vi "Adjust Min-Max.vi"(7 "log?":bool, 8 "error in (no error)":errorcluster, 9 "Secondary Graph":refnum<vi>, 10 "Primary Graph":refnum<vi>, 11 "Scan Driver.lvclass":refnum<class "Scan Driver.lvclass">) -> (0 "error out":errorcluster, 2 "High":dbl, 3 "Scan Driver.lvclass out":refnum<class "Scan Driver.lvclass">)   [LabVIEW 2012, in "Scan Driver.lvclass"]
doc: "Set the boundaries of the onscreen scan graphs according to the extrema of the data store."
uses:
  Scan Driver.lvclass
  Scan Driver.lvclass/Scan Driver.ctl
  Scanners/Scanner/Scanner.lvclass
  File IO/File IO.lvclass
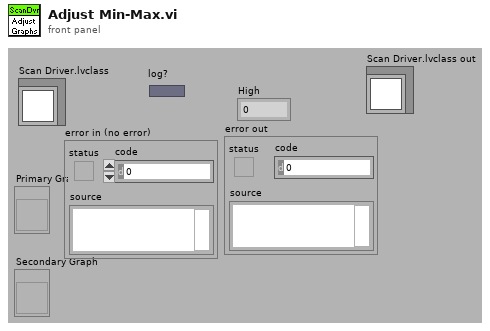
[diagram p1: front panel]
types:
  T1 = typedef "Readable.lvclass/Data Store.ctl" = T2[][]
  T2 = typedef "Readable.lvclass/Data Point.ctl" = cluster{"t":T3, "x":T4}
  T3 = typedef "Readable.lvclass/Time.ctl" = timestamp
  T4 = typedef "Readable.lvclass/X.ctl" = dbl
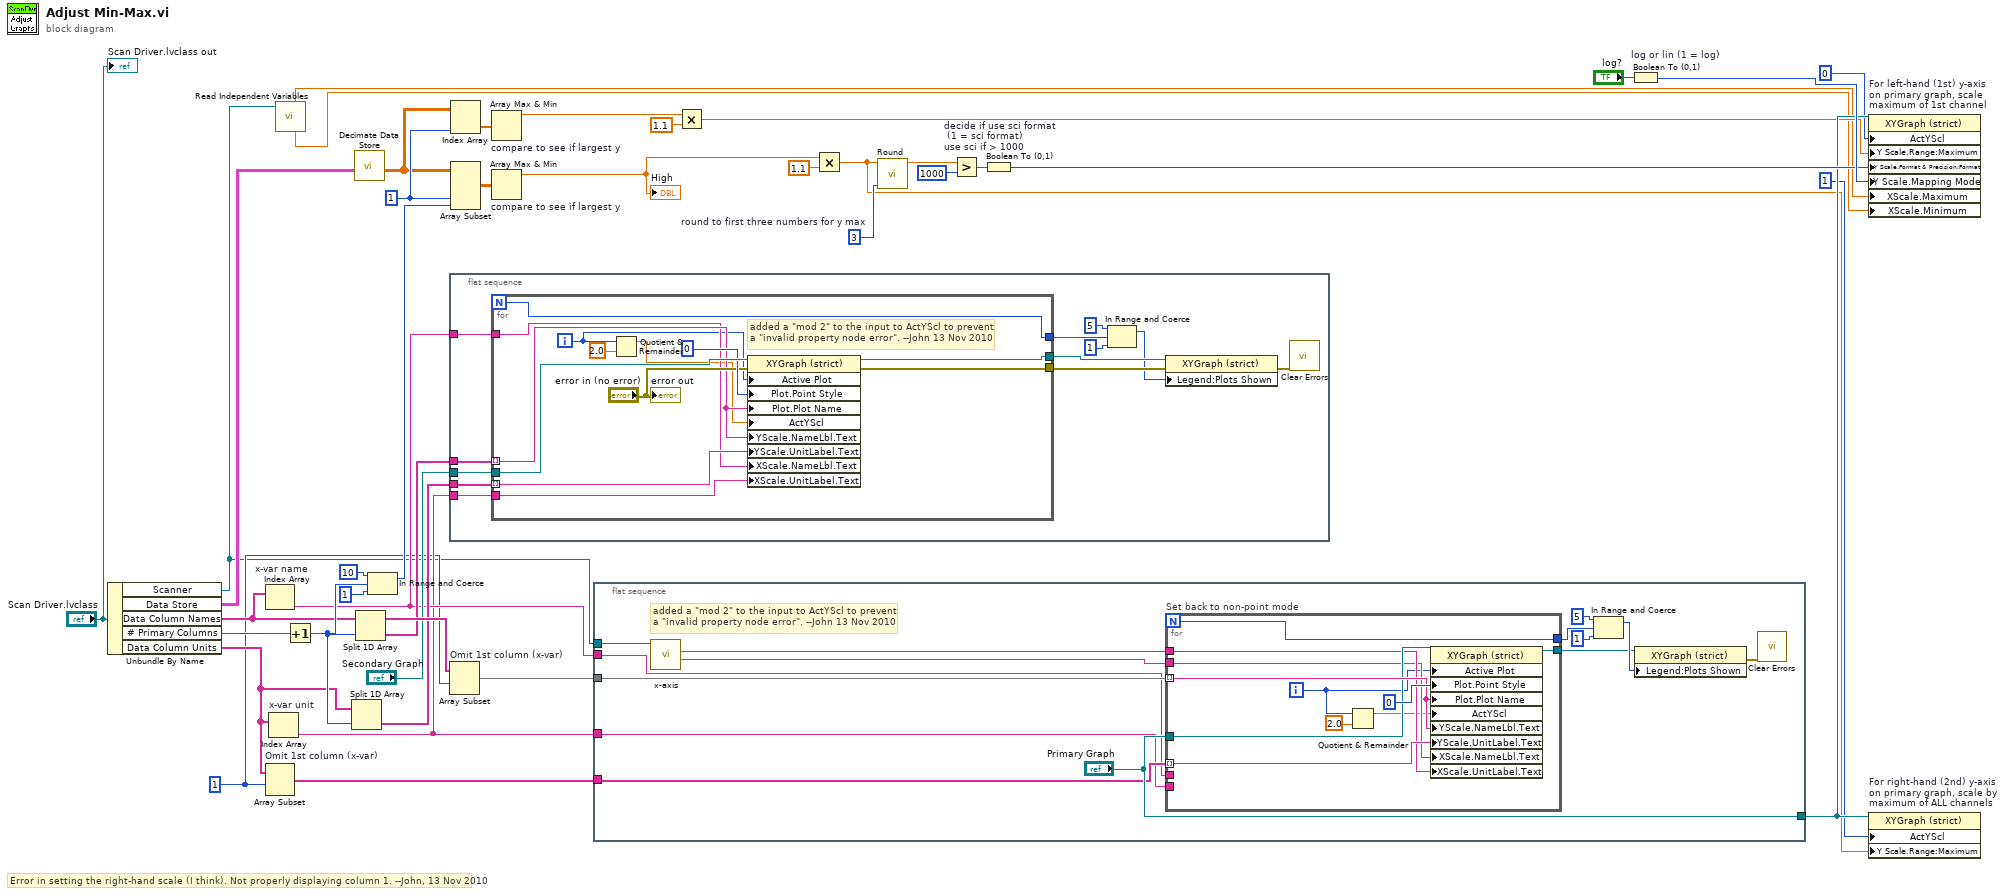
[diagram p0: block diagram]
diagram:
  w15 = 1 ("index")
  w9 = 1
  w24 = 3  # round to first three numbers for y max
  # "Error in setting the right-hand scale (I think). Not properly displaying column 1. --John, 13 Nov 2010"
  n1 = Unbundle By Name("Scan Driver.lvclass") -> ("Scanner"=w2:refnum<class "Scanner.lvclass">, "Data Store"=w10:T1, "Data Column Names"=w23:string[], "# Primary Columns"=w29:u32, "Data Column Units"=w22:string[])
  n2 = Index Array "x-var name"(array=w23) -> (element=w17:string)  [unwired: 1 in]
  n3 = Array Subset "Omit 1st column (x-var)"(array=w22, index=w15) -> (w18:string[])  [unwired: 1 in]
  n4 = Index Array "x-var unit"(array=w22) -> (element=w16:string)  [unwired: 1 in]
  n5 = call-dynamic "Read Independent Variables.vi"("Scanner.lvclass in"=w2) -> ("min value"=w4:dbl, "max value"=w3:dbl)  [unwired: 5 in, 4 out]
  n6 = Increment(x=w29) -> (x+1=w25:u32)
  n7 = Split 1D Array(array=w22, index=w25) -> (second subarray=w21:string[])  [unwired: 1 out]
  n8 = call "Decimate Data Store.vi"("Data Store"=w10) -> ("Data Points"=w1:T4[][])  [unwired: 9 in, 1 out]
  n9 = Split 1D Array(array=w23, index=w25) -> (first subarray=w28:string[], second subarray=w20:string[])
  n10 = In Range and Coerce(upper limit=u32 10, x=w25, lower limit=u32 1) -> (coerced(x)=w33:u32)  [unwired: 1 out]
  n11 = flat-sequence {
    tunnel: w21 -> [w46]
    tunnel: w20 -> [w45]
    tunnel: "Secondary Graph" -> [w44]
    tunnel: w17 -> [w43]
    tunnel: w16 -> [w42]
    frame #0 {
      n12 = for {
        N -> [w64]
        tunnel: w44 -> [w66]
        tunnel: w45 -> [w60] mode=indexing
        tunnel: [w64] -> w48
        tunnel: [w63] -> w53
        tunnel: [w61] -> w52
        tunnel: w46 -> [w59] mode=indexing
        tunnel: w43 -> [w58]
        tunnel: w42 -> [w57]
        i -> [w54]
        # "added a \"mod 2\" to the input to ActYScl to prevent a \"invalid property node error\". --John 13 Nov 2010"
        n13 = Quotient & Remainder(x=w54, y=2.0) -> (x-y*floor(x/y)=w55:dbl)  [unwired: 1 out]
        n14 = property on="Property Node" class="XYGraph (strict)"(reference=w66, error in="error in (no error)", "Active Plot"=w54, "Plot.Point Style"=0, "Plot.Plot Name"=w60, "ActYScl"=w55, "YScale.NameLbl.Text"=w60, "YScale.UnitLabel.Text"=w59, "XScale.NameLbl.Text"=w58, "XScale.UnitLabel.Text"=w57) -> (reference out=w63:refnum<vi>, error out=w61:errorcluster)
        "error out" <- "error in (no error)"
      }
      n15 = In Range and Coerce(upper limit=5, x=w48, lower limit=1) -> (coerced(x)=w47:i32)  [unwired: 1 out]
      n16 = property on="Property Node" class="XYGraph (strict)"(reference=w53, error in=w52, "Legend:Plots Shown"=w47) -> (error out=w51:errorcluster)  [unwired: 1 out]
      n17 = call <vilib>:"Clear Errors.vi"("error in (no error)"=w51) -> ()  [unwired: 6 in, 1 out]
    }
  }
  n18 = Array Subset "Omit 1st column (x-var)"(array=w28, index=w15) -> (w27:string[])  [unwired: 1 in]
  n19 = Index Array(array=w1, index (col)=w9) -> (element=w8:T4[])  [unwired: 1 in]
  n20 = Array Subset(array=w1, index (col)=w9, length (col)=w33) -> (w26:T4[][])  [unwired: 2 in]
  n21 = Array Max & Min "compare to see if largest y"(array=w8) -> (max value=w6:T4)  [unwired: 3 out]
  n22 = Array Max & Min "compare to see if largest y"(array=w26) -> (max value=w41:T4)  [unwired: 3 out]
  "High" <- w41
  n23 = flat-sequence {
    tunnel: w27 -> [w80]
    tunnel: ["Primary Graph"] -> w14
    tunnel: w18 -> [w73]
    tunnel: w17 -> [w72]
    tunnel: w16 -> [w71]
    tunnel: w2 -> [w69]
    frame #0 {
      # "added a \"mod 2\" to the input to ActYScl to prevent a \"invalid property node error\". --John 13 Nov 2010"
      n24 = call-dynamic "x-axis.vi"("Scanner in"=w69) -> ("Label"=w67:string, "Unit"=w68:string)  [unwired: 7 in, 2 out]
      n25 = for "Set back to non-point mode" {
        N -> [w91]
        tunnel: "Primary Graph" -> [w87]
        tunnel: w80 -> [w89] mode=indexing
        tunnel: [w91] -> w77
        tunnel: w73 -> [w88] mode=indexing
        tunnel: w72 -> [_]
        tunnel: w71 -> [_]
        tunnel: [w86] -> w70
        tunnel: w68 -> [w85]
        tunnel: w67 -> [w84]
        i -> [w81]
        n26 = Quotient & Remainder(x=w81, y=2.0) -> (x-y*floor(x/y)=w82:dbl)  [unwired: 1 out]
        n27 = property on="Property Node" class="XYGraph (strict)"(reference=w87, "Active Plot"=w81, "Plot.Point Style"=0, "Plot.Plot Name"=w89, "ActYScl"=w82, "YScale.NameLbl.Text"=w89, "YScale.UnitLabel.Text"=w88, "XScale.NameLbl.Text"=w84, "XScale.UnitLabel.Text"=w85) -> (reference out=w86:refnum<vi>)  [unwired: 1 in, 1 out]
      }
      n28 = In Range and Coerce(upper limit=5, x=w77, lower limit=1) -> (coerced(x)=w76:i32)  [unwired: 1 out]
      n29 = property on="Property Node" class="XYGraph (strict)"(reference=w70, "Legend:Plots Shown"=w76) -> (error out=w75:errorcluster)  [unwired: 1 in, 1 out]
      n30 = call <vilib>:"Clear Errors.vi"("error in (no error)"=w75) -> ()  [unwired: 6 in, 1 out]
    }
  }
  n31 = Multiply(x=w6, y=1.1) -> (x*y=w5:T4)
  n32 = Multiply(x=w41, y=1.1) -> (x*y=w12:T4)
  n33 = call "Round.vi"("place at this power of 10"=w24, "Number In"=w12) -> ("Number Out"=w30:dbl)  [unwired: 5 out]
  n34 = Greater?(x=w30, y=1000) -> (0:w36:bool)
  n35 = Boolean To (0,1) "decide if use sci format\n (1 = sci format)\nuse sci if > 1000"(Boolean=w36) -> (0, 1=w37:i16)
  n36 = Boolean To (0,1) "log or lin (1 = log)"(Boolean="log?") -> (0, 1=w38:i16)
  n37 = property on="For left-hand (1st) y-axis\non primary graph, scale\nmaximum of 1st channel" class="XYGraph (strict)"(reference=w14, "ActYScl"=0 ("Active Y Scale"), "Y Scale.Range:Maximum"=w5, "Y Scale.Format & Precision:Format"=w37, "Y Scale.Mapping Mode"=w38, "XScale.Maximum"=w3, "XScale.Minimum"=w4) -> ()  [unwired: 1 in, 2 out]
  n38 = property on="For right-hand (2nd) y-axis\non primary graph, scale by\nmaximum of ALL channels" class="XYGraph (strict)"(reference=w14, "ActYScl"=1 ("Active Y Scale"), "Y Scale.Range:Maximum"=w12) -> ()  [unwired: 1 in, 2 out]
  "Scan Driver.lvclass out" <- "Scan Driver.lvclass"
